vi "Get Voltage Step.vi"(8 "error in (no error)":errorcluster, 11 "Driver Test in":refnum<class "Driver Test.lvclass">) -> (0 "error out":errorcluster, 3 "Voltage Step":string)   [LabVIEW 2015, in "Driver Test.lvclass"]
doc: "Get the current voltage and dimming measurement step details. String is returned as \"[voltage]V_[dimming]Dimming\".\n\n<b>EXAMPLE</b>\n\"120V_10VDimming\""
uses:
  Driver Test.lvclass
  <vilib>/Cree, Inc/Cree Test Framework/Classes/Variable Engine/Class/Variable Engine.lvclass
  <vilib>/Cree, Inc/Cree Test Framework/Core Launcher/Core Launcher.lvlib
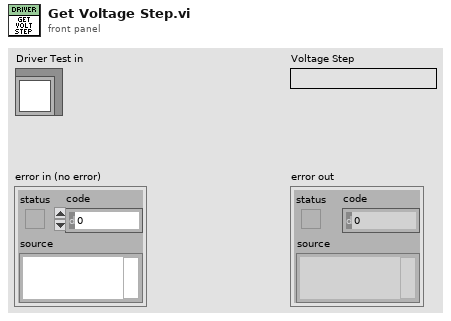
[diagram p1: front panel]
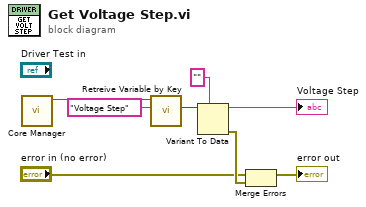
[diagram p0: block diagram]
diagram:
  n1 = call <vilib>:"Core Manager.vi"() -> ("Variable Engine"=w8:refnum<class "Variable Engine.lvclass">)  [unwired: 7 in, 4 out]
  n2 = call <vilib>:"Retreive Variable by Key.vi"("Key"="Voltage Step", "Acrobat Template in"=w8) -> ("Value"=w6:variant)  [unwired: 7 in, 2 out]
  n3 = Variant To Data(type="" ("Key"), Variant=w6) -> (data=→"Voltage Step":string, error out=w3:errorcluster)  [unwired: 1 in]
  n4 = Merge Errors("error in (no error)", w3) -> (→"error out":errorcluster)
